vi "Get Monotonically Increasing Item Name.vi"(8 "error in (no error)":errorcluster, 10 "Desired Name":string, 11 "Section Ptr":T1 format="%.0x") -> (0 "error out":errorcluster, 2 "New Item Name":string, 3 "Section Ptr out":T1 format="%.0x")   [LabVIEW 2020, in "Routing and Faulting System Explorer.lvlib"]
uses:
  Routing and Faulting System Explorer.lvlib
  <vilib>/NI VeriStand/Custom Device API/Custom Device Item Ref.ctl
  <vilib>/NI VeriStand/Custom Device API/Custom Device API.lvlib
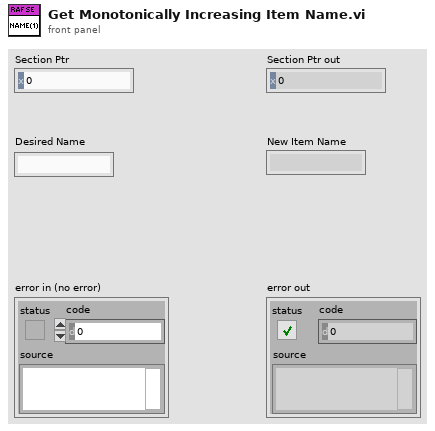
[diagram p1: front panel]
types:
  T1 = typedef "Custom Device API.lvlib/Custom Device Item Ref.ctl" = u64
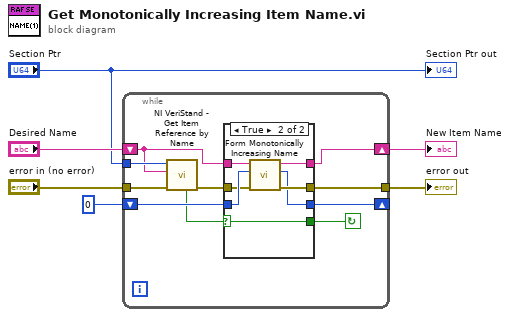
[diagram p0: block diagram]
diagram:
  n1 = while {
    tunnel: "error in (no error)" -> [w16]
    tunnel: "Section Ptr" -> [w15]
    shift-right: [w10] -> w3
    shift-left: "Desired Name" -> [w14]
    shift-right: [w11] -> _
    shift-left: 0 ("y") -> [w12]
    tunnel: [w8] -> w1
    stop <- w7 continue-if-true
    n2 = call <vilib>:"NI VeriStand - Get Item Reference by Name.vi"("error in (no error)"=w16, "Item Name"=w14, "Parent Ref in"=w15) -> ("error out"=w13:errorcluster, "Found"=w9:bool)  [unwired: 5 in, 2 out]
    n3 = case shown="True" w9 {
      selector: w9 -> [w17 w21]
      tunnel: w14 -> [w19 w26]
      tunnel: w13 -> [w18 w24]
      tunnel: w12 -> [w20 w27]
      tunnel: [w20 w22] -> w11
      tunnel: [w19 w25] -> w10
      tunnel: [w18 w23] -> w8
      tunnel: [w17 w21] -> w7
      frame False {
      }
      frame True {
        n4 = call "Form Monotonically Increasing Name.vi"("error in (no error)"=w24, "index"=w27, "Desired Name"=w26) -> ("error out"=w23:errorcluster, "next index"=w22:i32, "Next Candidate Name"=w25:string)  [unwired: 6 in]
      }
    }
  }
  "New Item Name" <- w3
  "error out" <- w1
  "Section Ptr out" <- "Section Ptr"
